vi "ingest.parquet_new_dataset.vi"(8 "error in":errorcluster, 11 "TabularIngestStaging in":refnum<class "TabularIngestStaging.lvclass">) -> (0 "error out":errorcluster, 3 "TabularIngestStaging out":refnum<class "TabularIngestStaging.lvclass">)   [LabVIEW 2020, in "TabularIngestStaging.lvclass"]
doc: "Ingests a Parquet file (or archive) into a newly created dataset."
uses:
  TabularIngestStaging.lvclass
  TabularIngestStaging.lvclass/TabularIngestStaging.ctl
  client.lvlib
panel:
  out "out_job out":i32
  in  "staging":i32
  in  "file_path":string
  in  "dataset_create":i32
  in  "out_job":i32
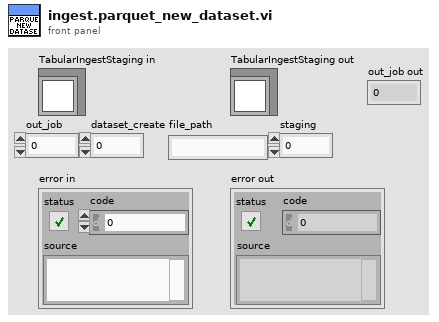
[diagram p1: front panel]
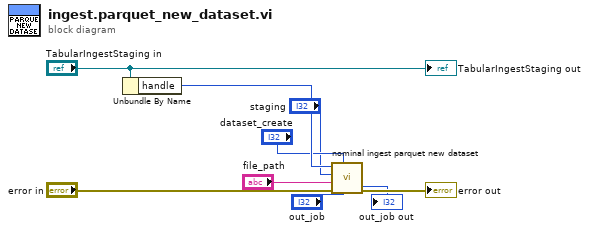
[diagram p0: block diagram]
diagram:
  n1 = Unbundle By Name("TabularIngestStaging in") -> ("handle"=w7:i32)
  n2 = call "nominal ingest parquet new dataset.vi"("out_job"="out_job", "dataset_create"="dataset_create", "error in (no error)"="error in", "file_path"="file_path", "staging"="staging", "client"=w7) -> ("error out"=→"error out":errorcluster, "out_job out"=→"out_job out":i32)  [unwired: 3 in, 1 out]
  "TabularIngestStaging out" <- "TabularIngestStaging in"
